vi "Main.vi"(8 "error in":errorcluster, 9 "Error Queue":refnum<queue>, 11 "Application Events":refnum<user-event>) -> (0 "error out":errorcluster)   [LabVIEW 2020, in "Error Handler.lvlib"]
doc: "VI Template with default error structure"
uses:
  Error Handler.lvlib
  Controls/Error Message Object.ctl
  Controller/Controls/Application Modules.ctl
  Controls/Error Commands.ctl
  Controller/Controls/Application Event Object.ctl
  Controller/Controls/Application Events.ctl
  Controls/Operational Loop Data.ctl
  Controls/Error Levels.ctl
  Controller/Controller.lvlib
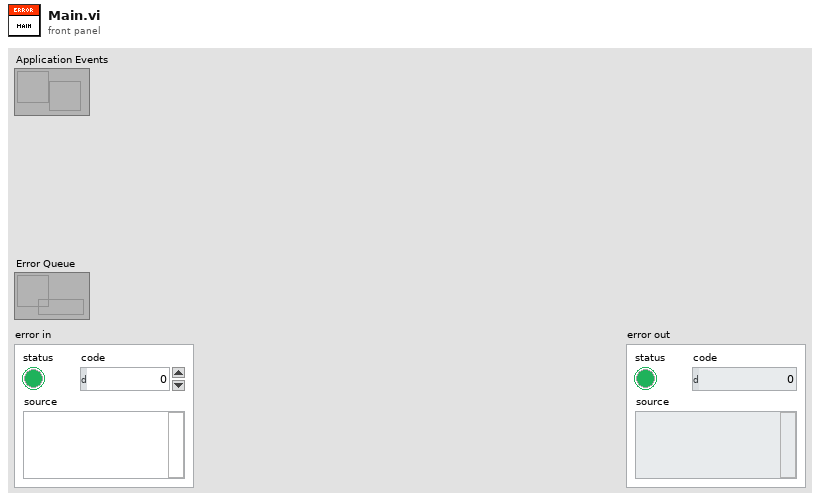
[diagram p1: front panel]
types:
  T1 = typedef "Error Handler.lvlib/Error Commands.ctl" = enum16{"Stop", "Process Error", "Initialize"}
  T2 = typedef "Error Handler.lvlib/Operational Loop Data.ctl" = cluster{"Error File":path}
  T3 = typedef "Controller.lvlib/Application Events.ctl" = enum16{"Terminate App", "Initialize", "New Transaction", "Balance Inquiry", "Deposit", "Withdrawal", "Fast Cash 50$", "Terminate Session", "Login", "Verify Account"}
  T4 = enum16{"Load References", "Release References", "Get References"}
  T5 = typedef "Controller.lvlib/Application Event Object.ctl" = cluster{"Events":T3, "Source Module":T6, "Event Data":variant}
  T6 = typedef "Controller.lvlib/Application Modules.ctl" = enum16{"Controller", "Error Module", "User Console", "Display Console", "Sensor Interface"}
  T7 = typedef "Error Handler.lvlib/Error Levels.ctl" = enum16{"Console Error", "Process Step Error", "Sensor Interface IO Error"}
  T8 = typedef "Error Handler.lvlib/Error Message Object.ctl" = cluster{"Source Module":T6, "Error":errorcluster, "Command":T9}
  T9 = typedef "Error Commands.ctl" = enum16{"Stop", "Process Error", "Initialize"}
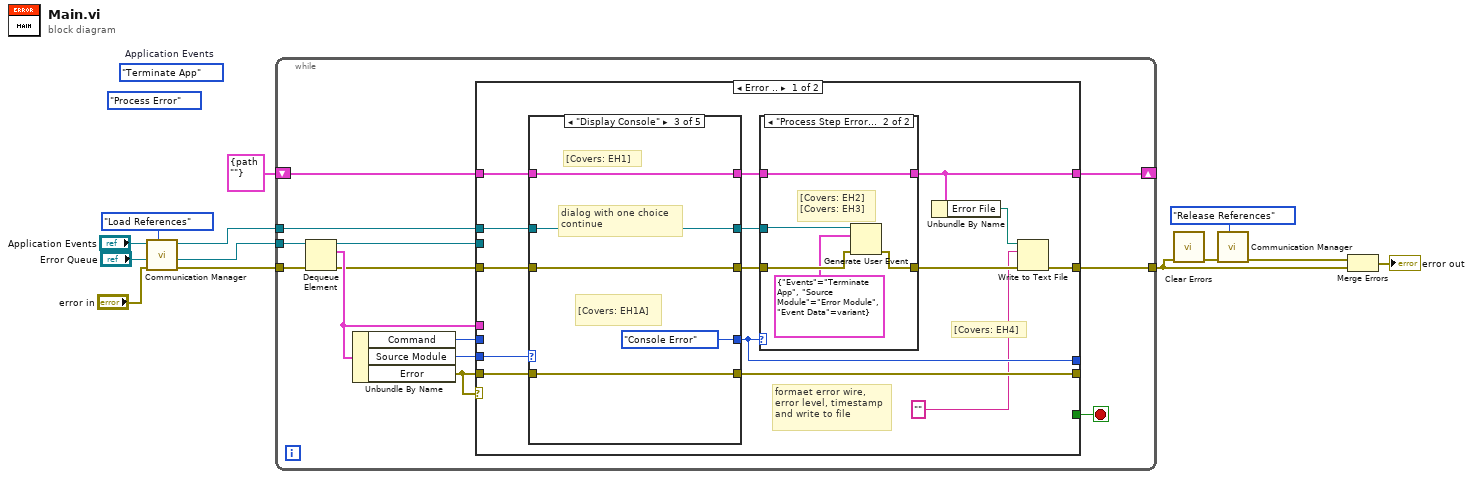
[diagram p0: block diagram]
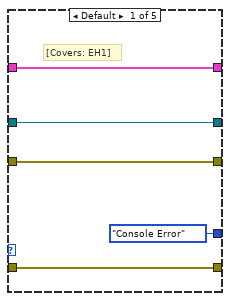
[diagram p3: hidden frame]
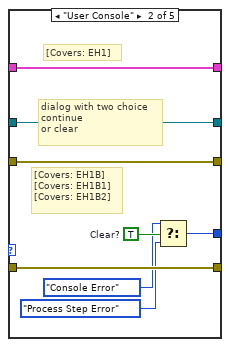
[diagram p4: hidden frame]
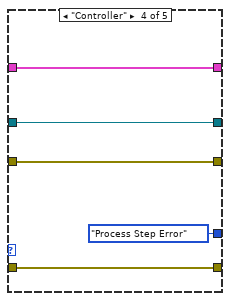
[diagram p5: hidden frame]
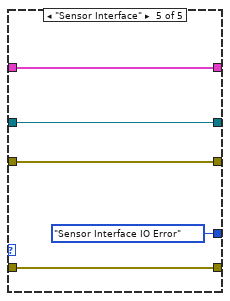
[diagram p6: hidden frame]
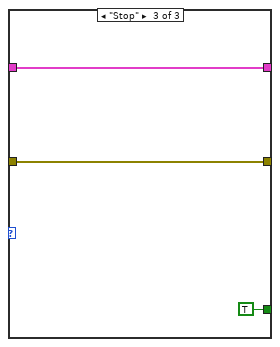
[diagram p9: hidden frame]
diagram:
  (unwired) Error_Commands."Process Error" ("Command")
  (unwired) Application_Events."Terminate App"  # Application Events
  n1 = call "Communication Manager.vi"("Mode"=T4."Load References", "error in"="error in", "Error Queue"="Error Queue", "Application Events"="Application Events") -> ("error out"=w10:errorcluster, "Error Queue Out"=w1:refnum<queue>, "Application Events Out"=w3:refnum<user-event>)  [unwired: 5 in]
  n2 = while {
    tunnel: w10 -> [w26]
    tunnel: w1 -> [w25]
    tunnel: [w24] -> w5
    tunnel: w3 -> [w20]
    shift-right: [w17] -> _
    shift-left: T2 {"Error File"=path ""} ("Operational Loop Data") -> [w18]
    stop <- w21 stop-if-true
    n3 = Dequeue Element(queue=w25, error in (no error)=w26) -> (queue out=w19:refnum<queue>, element=w23:T8, error out=w16:errorcluster)  [unwired: 1 in, 1 out]
    n4 = Unbundle By Name(w23) -> ("Command"=w14:T9, "Source Module"=w22:T6, "Error"=w15:errorcluster)
    n5 = case shown="Error .." w15 {
      tunnel: w16 -> [w40 w79]
      tunnel: [w30 w80] -> w24
      tunnel: w23 -> [_ _]
      tunnel: w22 -> [w37 _]
      tunnel: w15 -> [w34 _]
      tunnel: [_ w77] -> w21
      tunnel: w20 -> [w36 _]
      tunnel: w19 -> [_ _]
      tunnel: w18 -> [w41 w81]
      tunnel: [w28 w82] -> w17
      tunnel: w14 -> [_ w78]
      tunnel: [w33 _] -> _
      tunnel: [w32 _] -> _
      frame #0 {
        # "[Covers: EH4]"
        # "formaet error wire,\nerror level, timestamp\nand write to file"
        n6 = case shown="\"Display Console\"" w37 {
          tunnel: [w53 w61 w66 w71 w76] -> w39
          tunnel: w41 -> [w53 w61 w66 w71 w76]
          tunnel: [w52 w60 w65 w70 w75] -> w38
          tunnel: w40 -> [w52 w60 w65 w70 w75]
          tunnel: [Error_Levels."Console Error" ("Command") w56 Error_Levels."Console Error" ("Command") Error_Levels."Process Step Error" ("Command") Error_Levels."Sensor Interface IO Error" ("Command")] -> w32
          tunnel: w36 -> [w50 w59 w64 w68 w73]
          tunnel: [w50 w59 w64 w68 w73] -> w35
          tunnel: w34 -> [w49 w58 w63 w67 w72]
          tunnel: [w49 w58 w63 w67 w72] -> w33
          frame Default {
            # "[Covers: EH1]"
          }
          frame "User Console" {
            w57 = TRUE  # Clear?
            # "[Covers: EH1B] \n[Covers: EH1B1] \n[Covers: EH1B2]"
            # "dialog with two choice\ncontinue\nor clear"
            # "[Covers: EH1]"
            n7 = Select(t=Error_Levels."Console Error" ("Command"), s=w57, f=Error_Levels."Process Step Error" ("Command")) -> (s? t:f=w56:T7)
          }
          frame "Display Console" {
            # "[Covers: EH1A]"
            # "dialog with one choice\ncontinue"
            # "[Covers: EH1]"
          }
          frame "Controller" {
          }
          frame "Sensor Interface" {
          }
        }
        n8 = case shown="\"Process Step Error\", \"Sensor Interface IO Error\"" w32 {
          tunnel: [w43 w48] -> w28
          tunnel: w39 -> [w43 w48]
          tunnel: [w42 w45] -> w31
          tunnel: w38 -> [w42 w46]
          tunnel: w35 -> [_ w47]
          frame Default {
          }
          frame "Process Step Error", "Sensor Interface IO Error" {
            # "[Covers: EH2] \n[Covers: EH3]"
            n9 = Generate User Event(user event=w47, event data cluster=T5 {"Events"=enum."Terminate App", "Source Module"=enum."Error Module", "Event Data"=variant} ("event data"), error in=w46) -> (error out=w45:errorcluster)  [unwired: 1 in, 1 out]
          }
        }
        n10 = Unbundle By Name(w28) -> ("Error File"=w27:path)
        n11 = Write to Text File(file (use dialog)=w27, text="", error in=w31) -> (error out=w30:errorcluster)  [unwired: 1 in, 2 out]
      }
      frame #1 {
        n12 = case shown="Default" w78 {
          tunnel: [w84 w86 w89] -> w82
          tunnel: w81 -> [w84 w86 w89]
          tunnel: [w83 w85 w88] -> w80
          tunnel: w79 -> [w83 w85 w88]
          tunnel: [_ _ TRUE] -> w77
          frame Default {
          }
          frame "Initialize" {
            # "create error file \nstore path"
          }
          frame "Stop" {
          }
        }
      }
    }
  }
  n13 = call <vilib>:"Clear Errors.vi"("error in (no error)"=w5) -> ("error out"=w8:errorcluster)  [unwired: 5 in, 1 out]
  n14 = call "Communication Manager.vi"("Mode"=T4."Release References", "error in"=w8) -> ("error out"=w4:errorcluster)  [unwired: 7 in, 2 out]
  n15 = Merge Errors(w4, w5) -> (→"error out":errorcluster)
